vi "graph 1.vi"(9 "phase":dbl format="%.2p", 10 "amplitude":dbl=1.0 format="%0.2p") -> (2 "Waveform Graph":waveform(dbl)(graph))   [LabVIEW 2025]
uses:
  <vilib>/measure/NI_MABase.lvlib
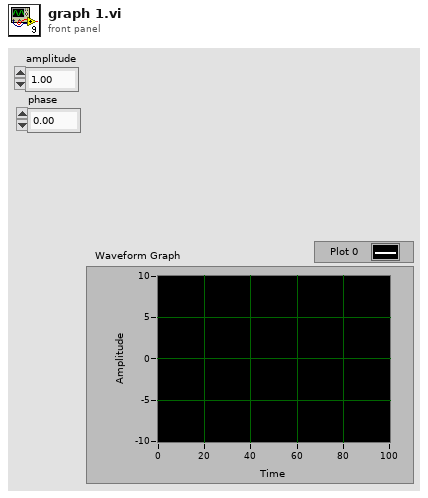
[diagram p1: front panel]
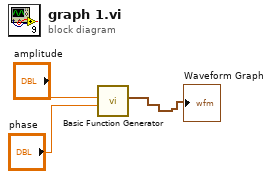
[diagram p0: block diagram]
diagram:
  n1 = call <vilib>:"Basic Function Generator.vi"("phase"="phase", "amplitude"="amplitude") -> ("signal out"=→"Waveform Graph":waveform(dbl))  [unwired: 7 in, 2 out]
